vi "Is LVUnit Test.vi"(11 "ProjectItem Refnum":refnum<vi>) -> (2 "Is LVUnit Test":bool)   [LabVIEW 2017, in "LVUnit Test Discoverer.lvclass"]
uses:
  LVUnit Test Discoverer.lvclass
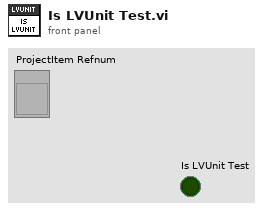
[diagram p1: front panel]
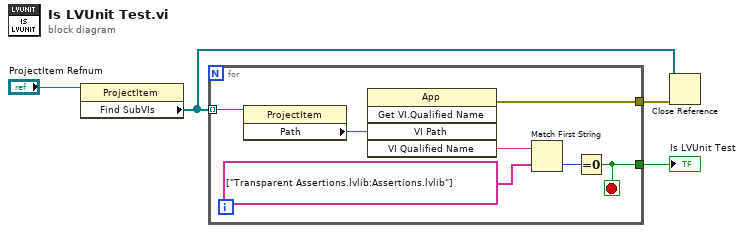
[diagram p0: block diagram]
diagram:
  n1 = property class="ProjectItem"(reference="ProjectItem Refnum") -> ("Find SubVIs"=w1:refnum<vi>[])  [unwired: 1 in, 2 out]
  n2 = for {
    tunnel: w1 -> [w11] mode=indexing
    tunnel: [w6] -> w3
    tunnel: [w5] -> w2
    stop <- w6 stop-if-true
    n3 = property class="ProjectItem"(reference=w11) -> ("Path"=w10:path)  [unwired: 1 in, 2 out]
    n4 = invoke class="App" method="Get VI.Qualified Name"("VI Path"=w10) -> (error out=w5:errorcluster, "VI Qualified Name"=w9:string)  [unwired: 4 in, 3 out]
    n5 = Match First String(2:string[] ["Transparent Assertions.lvlib:Assertions.lvlib"] ("string array"), 3:w9) -> (0:w7:i32)  [unwired: 1 out]
    n6 = Equal To 0?(x=w7) -> (x = 0?=w6:bool)
  }
  "Is LVUnit Test" <- w3
  n7 = Close Reference(reference=w1, error in (no error)=w2) -> ()  [unwired: 1 out]
